vi "Get Site Ref Mic Data.vi"(0 "Site Number":i32, 11 "error in (no error)":errorcluster) -> (4 "Serial Number":u32, 6 "Ref Mic Sensitivity (mV/Pa)":dbl, 8 "Ref Mic Cal File Data":string[][](array[string]), 15 "error out":errorcluster)   [LabVIEW 2020]
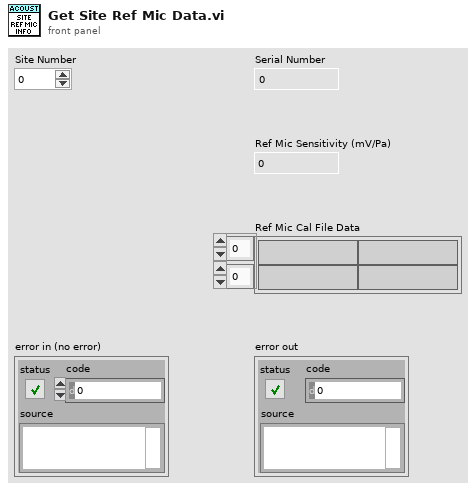
[diagram p1: front panel]
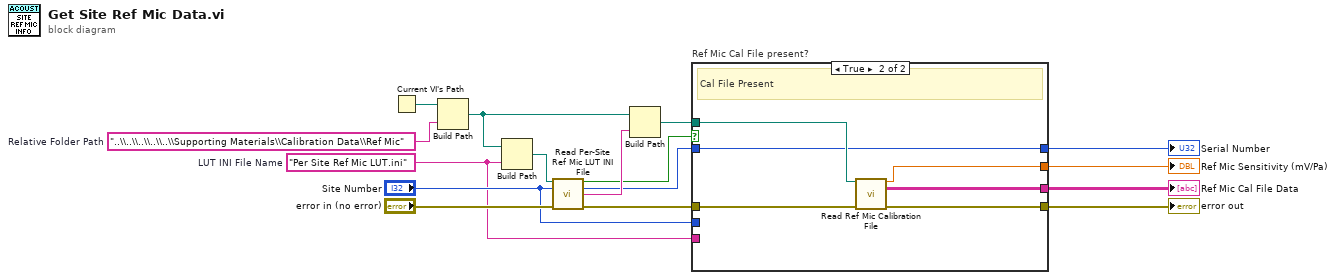
[diagram p0: block diagram]
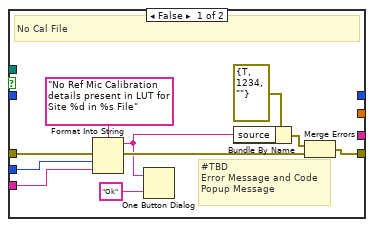
[diagram p2: hidden frame]
diagram:
  w2 = "Per Site Ref Mic LUT.ini"  # LUT INI File Name
  w6 = "..\\..\\..\\..\\..\\Supporting Materials\\Calibration Data\\Ref Mic"  # Relative Folder Path
  n1 = Current VI's Path() -> (path=w7:path)
  n2 = Build Path(base path=w7, name or relative path=w6) -> (appended path=w5:path)
  n3 = Build Path(base path=w5, name or relative path=w2) -> (appended path=w4:path)
  n4 = call "Read Per-Site Ref Mic LUT INI File.vi"("LUT INI File Path"=w4, "Site Number"="Site Number", "error in (no error)"="error in (no error)") -> ("Found?"=w10:bool, "Serial Number"=w9:u32, "Calibration File Name"=w14:string, "error out"=w15:errorcluster)  [unwired: 9 in]
  n5 = Build Path(base path=w5, name or relative path=w14) -> (appended path=w13:path)
  n6 = case "Ref Mic Cal File present?" shown="True" w10 {
    tunnel: w15 -> [w26 w32]
    tunnel: w13 -> [_ w31]
    tunnel: [w20 w30] -> w12
    tunnel: [_ w29] -> w11
    tunnel: w9 -> [_ w28]
    tunnel: [_ w28] -> w8
    tunnel: "Site Number" -> [w23 _]
    tunnel: w2 -> [w22 _]
    tunnel: [_ w27] -> w1
    frame False {
      # "#TBD\nError Message and Code\nPopup Message"
      # "No Cal File"
      n7 = Format Into String(format string="No Ref Mic Calibration details present in LUT for Site %d in %s File", error in=w26, w23, w22) -> (resulting string=w17:string, error out=w24:errorcluster)  [unwired: 1 in]
      n8 = One Button Dialog(message=w17, button name ("OK")="Ok") -> ()  [unwired: 1 out]
      n9 = Bundle By Name(cluster=errorcluster {"status"=TRUE, "code"=1234, "source"=""} ("error in"), "source"=w17) -> (w18:errorcluster)
      n10 = Merge Errors(w18, w24) -> (w20:errorcluster)
    }
    frame True {
      # "Cal File Present"
      n11 = call "Read Ref Mic Calibration File.vi"("Calibration File Path"=w31, "error in (no error)"=w32) -> ("Sensitivity (mV/Pa)"=w29:dbl, "Ref Mic Cal File Data"=w27:string[][], "error out"=w30:errorcluster)  [unwired: 11 in]
    }
  }
  "error out" <- w12
  "Ref Mic Sensitivity (mV/Pa)" <- w11
  "Serial Number" <- w8
  "Ref Mic Cal File Data" <- w1
